vi "Desktop Main.vi"() -> ()   [LabVIEW 2015]
uses:
  <vilib>/FPGAPlugInAG/Digital Systems Development Board/niLvFpga_Open_Digital Systems Development Board.vi
  <vilib>/Utility/error.llb/Error Cluster From Error Code.vi
  <vilib>/rvi/errors/niLvFpgaAdjustHostInterfaceError.vi
  <vilib>/rvi/interface/nirviOpenFPGA/nirviOpenFPGA.xnode
  FPGA Bitfiles/Audio_FPGATarget_FPGAMain_3psOd07Wy8k.lvbitx
  FPGA Main.vi
  <vilib>/rvi/interface/nirviReadWriteControl/nirviReadWriteControl.xnode
  Desktop Sub VIs/DSDB FPGA Ref.ctl
  resource/NiAdept/NiAdept.dll
panel:
  in  "I2S.MUTEN":bool=TRUE
  in  "I2S.BitCount":u16=32
  in  "I2S.WordLength":u16=32
  in  "Analog Bypass":bool
  in  "SSM2603 Register":cluster{"Addr":u8, "Data":u16}[](array[cluster])=[{"Addr"=0, "Data"=23}, {"Addr"=1, "Data"=23}, {"Addr"=2, "Data"=116}, {"Addr"=3, "Data"=116}, {"Addr"=4, "Data"=16}, {"Addr"=5, "Data"=0}, {"Addr"=7, "Data"=14}, {"Addr"=8, "Data"=28}] {"Data" format="b%09b"}
  in  "Digital Bypass":bool
  in  "Reset":bool
  out "error out":errorcluster
  in  "stop":bool
  # "Overview: This VI demostrates how to control the DSDB audio module and implement bypass function.\nRequirements: LabVIEW FPGA Module, Xilinx Compilation Tools for Vivado, LabVIEW Support for Digital Systems Development Board\nInstructions:\n1. Make sure the FPGA Main.vi has been built.\n2. Connect an audio output signal to Line In jack, and connect headphone to HPH Out jack.\n3. Click Reset button to reset audio chip's configuration.\n4. Click Digital Bypass button, and then the audio signal will be played through headphone.\n5. Click Analog Bypass button, and the result should be similar with Digital Bypass mode."
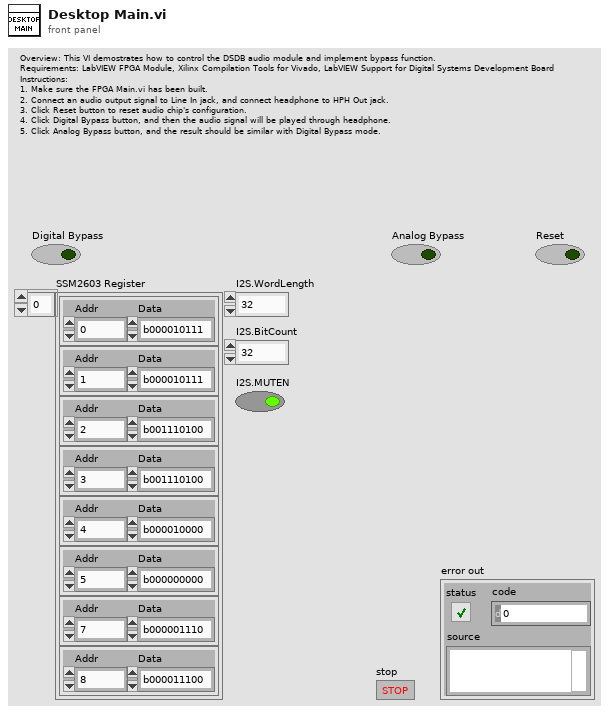
[diagram p1: front panel]
types:
  T1 = typedef "DSDB FPGA Ref.ctl" = refnum<k20>
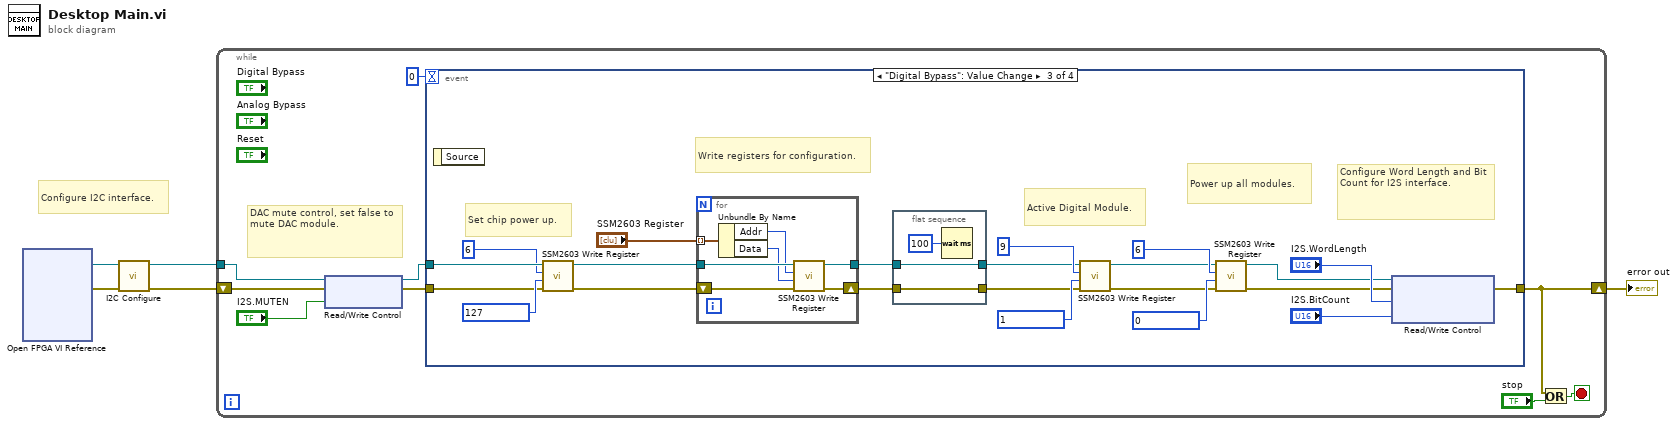
[diagram p0: block diagram]
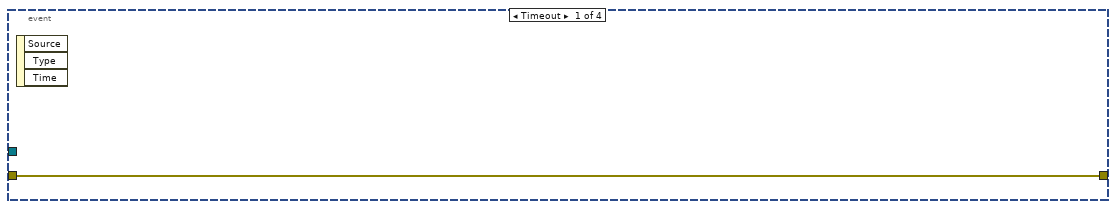
[diagram p2: hidden frame]
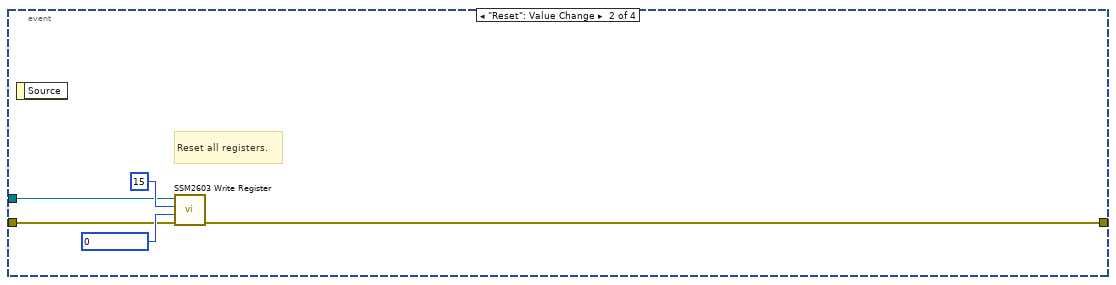
[diagram p3: hidden frame]
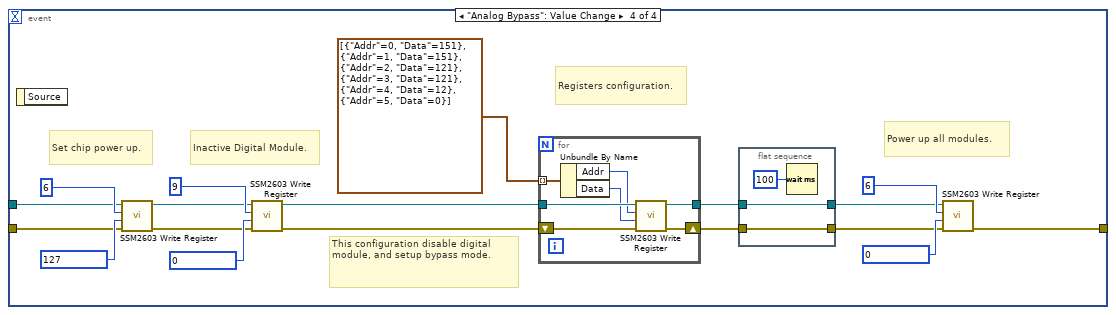
[diagram p4: hidden frame]
diagram:
  # "Configure I2C interface."
  n1 = xnode "Open FPGA VI Reference"() -> ("FPGA VI Reference Out"=w3:refnum<k20>, "error out"=w5:errorcluster)  [unwired: 2 in]
  n2 = call "I2C Configure.vi"("error in"=w5, "FPGA VI Reference In"=w3) -> ("error out"=w2:errorcluster, "FPGA VI Reference Out"=w1:T1)  [unwired: 8 in]
  n3 = while {
    tunnel: w1 -> [w8]
    shift-right: [w11] -> w4
    shift-left: w2 -> [w9]
    stop <- w14 stop-if-true
    # "DAC mute control, set false to mute DAC module."
    n4 = xnode "Read/Write Control"("FPGA VI Reference In"=w8, "error in"=w9, "I2S.MUTEN"="I2S.MUTEN") -> ("FPGA VI Reference Out"=w7:T1, "error out"=w10:errorcluster)
    n5 = event shown="[2] \"Digital Bypass\": Value Change" {
      selector: _ -> [_ _ _ _]
      dyn-events: _ -> [_ _ _ _]
      timeout: 0 -> [_ _ _ _]
      tunnel: w7 -> [_ w18 w24 w67]
      tunnel: w10 -> [w15 w17 w25 w52]
      tunnel: [w15 w16 w31 w62] -> w11
      event Timeout {
        n6 = event-data() -> ()  [unwired: 1 in, 3 out]
      }
      event "Reset": Value Change {
        # "Reset all registers."
        n7 = event-data() -> ()  [unwired: 1 in, 1 out]
        n8 = call "SSM2603 Write Register.vi"("Error In (No Error)"=w17, "Reg Data"=u16 0, "Reg Address"=u8 15, "FPGA VI Reference In"=w18) -> ("error out"=w16:errorcluster)  [unwired: 6 in, 1 out]
      }
      event "Digital Bypass": Value Change {
        # "Configure Word Length and Bit Count for I2S interface."
        # "Power up all modules."
        # "Active Digital Module."
        # "Write registers for configuration."
        # "Set chip power up."
        n9 = event-data() -> ()  [unwired: 1 in, 1 out]
        n10 = call "SSM2603 Write Register.vi"("Error In (No Error)"=w25, "Reg Data"=u16 127, "Reg Address"=u8 6, "FPGA VI Reference In"=w24) -> ("error out"=w21:errorcluster, "FPGA VI Reference Out"=w22:T1)  [unwired: 6 in]
        n11 = for {
          tunnel: w22 -> [w50]
          shift-right: [w45] -> w28
          shift-left: w21 -> [w51]
          tunnel: "SSM2603 Register" -> [w49] mode=indexing
          tunnel: [w46] -> w30
          n12 = Unbundle By Name(w49) -> ("Addr"=w48:u8, "Data"=w47:u16)
          n13 = call "SSM2603 Write Register.vi"("Error In (No Error)"=w51, "Reg Data"=w47, "Reg Address"=w48, "FPGA VI Reference In"=w50) -> ("error out"=w45:errorcluster, "FPGA VI Reference Out"=w46:T1)  [unwired: 6 in]
        }
        n14 = flat-sequence {
          tunnel: [w43] -> _
          tunnel: w30 -> [w42]
          tunnel: w28 -> [w43]
          tunnel: [w42] -> w29
          frame #0 {
            n15 = Wait (ms)(milliseconds to wait=u32 100) -> ()  [unwired: 1 out]
          }
        }
        n16 = call "SSM2603 Write Register.vi"("Error In (No Error)"=w28, "Reg Data"=u16 1, "Reg Address"=u8 9, "FPGA VI Reference In"=w29) -> ("error out"=w26:errorcluster, "FPGA VI Reference Out"=w27:T1)  [unwired: 6 in]
        n17 = call "SSM2603 Write Register.vi"("Error In (No Error)"=w26, "Reg Data"=u16 0, "Reg Address"=u8 6, "FPGA VI Reference In"=w27) -> ("error out"=w34:errorcluster, "FPGA VI Reference Out"=w35:T1)  [unwired: 6 in]
        n18 = xnode "Read/Write Control"("FPGA VI Reference In"=w35, "error in"=w34, "I2S.WordLength"="I2S.WordLength", "I2S.BitCount"="I2S.BitCount") -> ("error out"=w31:errorcluster)  [unwired: 1 out]
      }
      event "Analog Bypass": Value Change {
        # "This configuration disable digital module, and setup bypass mode."
        # "Registers configuration."
        # "Power up all modules."
        # "Inactive Digital Module."
        # "Set chip power up."
        n19 = event-data() -> ()  [unwired: 1 in, 1 out]
        n20 = call "SSM2603 Write Register.vi"("Error In (No Error)"=w52, "Reg Data"=u16 127, "Reg Address"=u8 6, "FPGA VI Reference In"=w67) -> ("error out"=w58:errorcluster, "FPGA VI Reference Out"=w59:T1)  [unwired: 6 in]
        n21 = call "SSM2603 Write Register.vi"("Error In (No Error)"=w58, "Reg Data"=u16 0, "Reg Address"=u8 9, "FPGA VI Reference In"=w59) -> ("error out"=w60:errorcluster, "FPGA VI Reference Out"=w61:T1)  [unwired: 6 in]
        n22 = for {
          tunnel: w61 -> [w75]
          shift-right: [w70] -> w57
          shift-left: w60 -> [w76]
          tunnel: cluster{"Addr":u8, "Data":u16}[] [{"Addr"=0, "Data"=151}, {"Addr"=1, "Data"=151}, {"Addr"=2, "Data"=121}, {"Addr"=3, "Data"=121}, {"Addr"=4, "Data"=12}, {"Addr"=5, "Data"=0}] ("SSM2603 Register") -> [w74] mode=indexing
          tunnel: [w71] -> w55
          n23 = Unbundle By Name(w74) -> ("Addr"=w73:u8, "Data"=w72:u16)
          n24 = call "SSM2603 Write Register.vi"("Error In (No Error)"=w76, "Reg Data"=w72, "Reg Address"=w73, "FPGA VI Reference In"=w75) -> ("error out"=w70:errorcluster, "FPGA VI Reference Out"=w71:T1)  [unwired: 6 in]
        }
        n25 = flat-sequence {
          tunnel: w57 -> [w78]
          tunnel: w55 -> [w77]
          tunnel: [w78] -> w56
          tunnel: [w77] -> w54
          frame #0 {
            n26 = Wait (ms)(milliseconds to wait=u32 100) -> ()  [unwired: 1 out]
          }
        }
        n27 = call "SSM2603 Write Register.vi"("Error In (No Error)"=w56, "Reg Data"=u16 0, "Reg Address"=u8 6, "FPGA VI Reference In"=w54) -> ("error out"=w62:errorcluster)  [unwired: 6 in, 1 out]
      }
    }
    n28 = Or(x=w11, y="stop") -> (x .or. y?=w14:bool)
  }
  "error out" <- w4
